vi "Run cmd File.vi"(7 "wait until completion? (T)":bool=TRUE, 8 "Error in":errorcluster caption="Error in (no error)", 10 "args":string[](array[string]), 11 "name or relative path":string="Open_dir_in_VSCode.cmd") -> (0 "Error out":errorcluster, 2 "before substring":string="cmd /c \"D:\\OneDrive\\Projects\\Libraries\\NEVSTOP-LAB\\SimpleGit-Provider\\SimpleGit\\Git\\_scripts\\Open_dir_in_VSCode.cmd\" D:\\OneDrive\\Projects\\Libraries\\NEVSTOP-LAB\\SimpleGit-Provider", 3 "standard output":string)   [LabVIEW 2017]
panel:
  # "Check_if_totoisegit_installed.cmd"
  # "Check_if_vscode_installed.cmd"
  # "D:\\1 2 3"
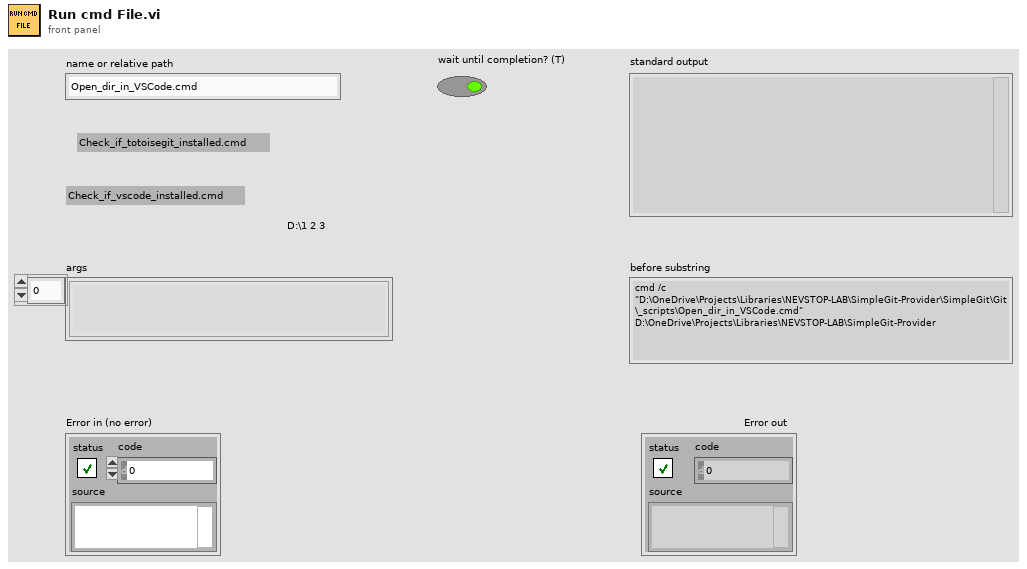
[diagram p1: front panel]
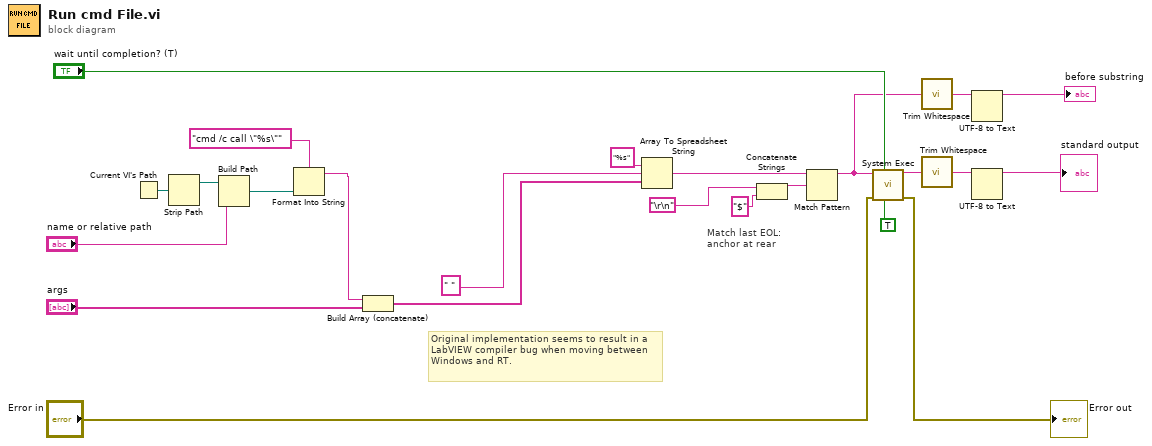
[diagram p0: block diagram]
diagram:
  # "Original implementation seems to result in a LabVIEW compiler bug when moving between Windows and RT."
  # "Match last EOL:\nanchor at rear"
  n1 = Current VI's Path() -> (path=w21:path)
  n2 = Strip Path(path=w21) -> (stripped path=w20:path)  [unwired: 1 out]
  n3 = Build Path(base path=w20, name or relative path="name or relative path") -> (appended path=w19:path)
  n4 = Format Into String(format string="cmd /c call \"%s\"", w19) -> (resulting string=w14:string)  [unwired: 2 in, 1 out]
  n5 = Build Array (concatenate)(w14, "args") -> (w15:string[])
  n6 = Array To Spreadsheet String(delimiter (Tab)=" ", array=w15, 3:"%s" ("format string")) -> (spreadsheet string=w12:string)
  n7 = Concatenate Strings("\r\n", "$" ("Substring")) -> (w11:string)
  n8 = Match Pattern(string=w12, regular expression=w11) -> (before substring=w3:string)  [unwired: 1 in, 3 out]
  n9 = call <vilib>:"System Exec.vi"("run minimized? (F)"=TRUE, "wait until completion? (T)"="wait until completion? (T)", "error in (no error)"="Error in", "command line"=w3) -> ("error out"=→"Error out":errorcluster, "standard output"=w4:string)  [unwired: 4 in, 2 out]
  n10 = call <vilib>:"Trim Whitespace.vi"("string"=w3) -> ("trimmed string"=w1:string)  [unwired: 1 in]
  n11 = call <vilib>:"Trim Whitespace.vi"("string"=w4) -> ("trimmed string"=w2:string)  [unwired: 1 in]
  n12 = UTF-8 to Text(11:w1) -> (3:→"before substring":string)  [unwired: 2 in, 1 out]
  n13 = UTF-8 to Text(11:w2) -> (3:→"standard output":string)  [unwired: 2 in, 1 out]
